vi "Database_UUT_Create.vi"(0 "reference in":refnum<class "Database_UUT.lvclass">, 5 "error in (no error)":errorcluster) -> (14 "reference out":refnum<class "Database_UUT.lvclass">, 19 "error out":errorcluster)   [LabVIEW 2017, in "Database_UUT.lvclass"]
uses:
  Database_UUT.lvclass
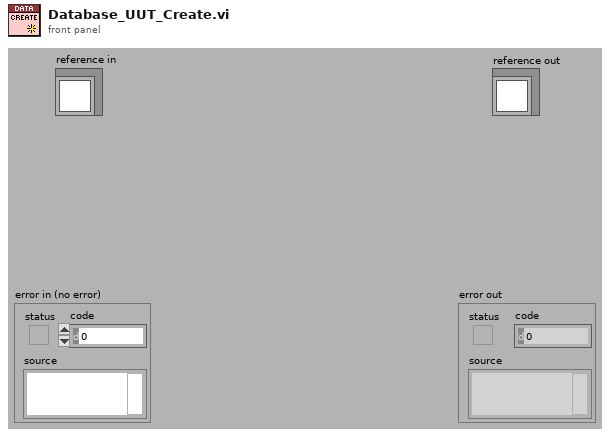
[diagram p1: front panel]
types:
  T1 = typedef "Database.lvclass/ObjectAttributes.ctl" = cluster{"Filepath to Database":path}
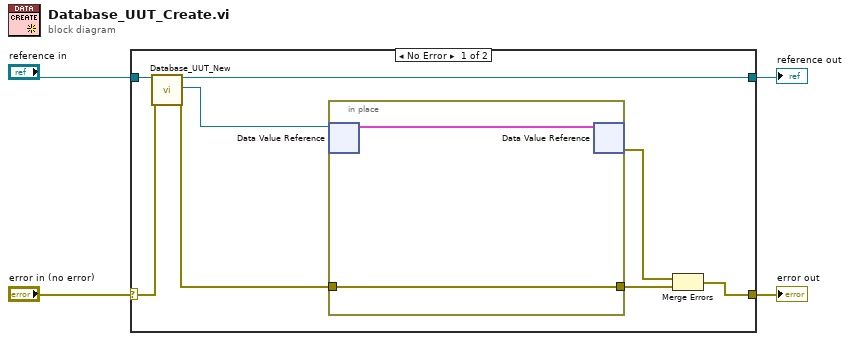
[diagram p0: block diagram]
diagram:
  n1 = case shown="No Error" "error in (no error)" {
    selector: "error in (no error)" -> [w11 w16]
    tunnel: [w8 w16] -> w3
    tunnel: "reference in" -> [w12 w15]
    tunnel: [w10 w15] -> w1
    frame No Error {
      n2 = call "Database_UUT_New.vi"("reference in"=w12, "error in (no error)"=w11) -> ("reference out"=w10:refnum<class "Database_UUT.lvclass">, "DVRRefOut"=w7:refnum<data-value>, "error out"=w6:errorcluster)  [unwired: 14 in, 1 out]
      n3 = in-place {
        in-place-border: w6 -> [w14]
        in-place-border: [w14] -> w5
        n4 = in-place-dvr #1(w7) -> (w13:T1)  [unwired: 1 out]
        n5 = in-place-dvr #1(w13) -> (w9:errorcluster)  [unwired: 1 out]
      }
      n6 = Merge Errors(w9, w5) -> (w8:errorcluster)
    }
    frame Error {
    }
  }
  "error out" <- w3
  "reference out" <- w1
